vi "Fetch (NT Enum (Index).vi"(6 "default timestamp":timestamp, 7 "PV name":string, 8 "error in":errorcluster, 10 "default index":u16, 11 "Server in":refnum<class "Server.lvclass">) -> (0 "error out":errorcluster, 1 "PV found?":bool, 2 "index":u16, 3 "Server out":refnum<class "Server.lvclass">, 4 "timestamp":timestamp)   [LabVIEW 2020, in "PV Access.lvlib" / "PVA Server.lvlib" / "Server.lvclass"]
uses:
  Server.lvclass
  PV Data/PV Data/PV Data.lvclass
  Source/Source.lvclass
  Server.lvclass/Server.ctl
  PV Data/PV Data/Read Field (U16).vi
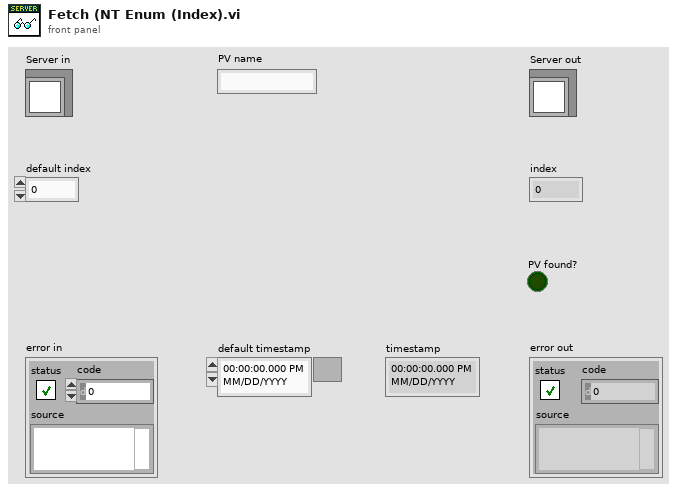
[diagram p1: front panel]
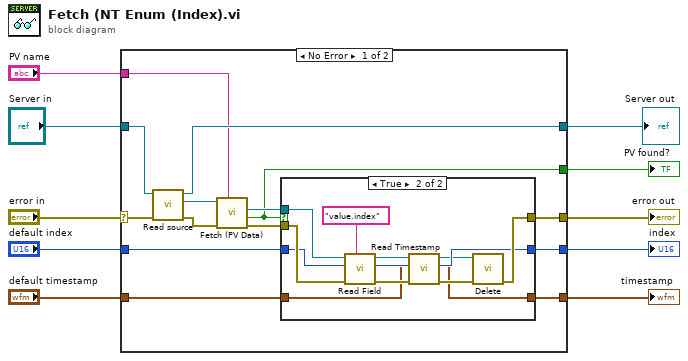
[diagram p0: block diagram]
diagram:
  n1 = case shown="No Error" "error in" {
    selector: "error in" -> [w12 w41]
    tunnel: [w17 w41] -> w10
    tunnel: "PV name" -> [w21 _]
    tunnel: "Server in" -> [w23 w43]
    tunnel: [w22 w43] -> w6
    tunnel: "default index" -> [w16 w42]
    tunnel: [w15 w42] -> w4
    tunnel: "default timestamp" -> [w14 w40]
    tunnel: [w13 w40] -> w2
    tunnel: [w11 _] -> w1
    frame No Error {
      n2 = call "Read source.vi"("error in (no error)"=w12, "Server in"=w23) -> ("error out"=w20:errorcluster, "Source"=w19:refnum<class "Source.lvclass">, "Server out"=w22:refnum<class "Server.lvclass">)  [unwired: 7 in]
      n3 = call "Fetch (PV Data).vi"("PV name"=w21, "error in"=w20, "Source in"=w19) -> ("error out"=w24:errorcluster, "PV found?"=w11:bool, "PV Data out"=w18:refnum<class "PV Data.lvclass">)  [unwired: 5 in, 1 out]
      n4 = case shown="True" w11 {
        tunnel: w24 -> [w26 w39]
        tunnel: w18 -> [_ w38]
        tunnel: [w26 w37] -> w17
        tunnel: w16 -> [w25 w36]
        tunnel: [w25 w32] -> w15
        tunnel: w14 -> [w27 w29]
        tunnel: [w27 w28] -> w13
        frame False {
        }
        frame True {
          n5 = call-poly "Read Field.vi"("field name"="value.index", "error in (no error)"=w39, "default"=w36, "PV Data in"=w38) -> ("error out"=w34:errorcluster, "value"=w32:u16, "PV Data out"=w33:refnum<class "PV Data.lvclass">)  [unwired: 5 in]
          n6 = call "Read Timestamp.vi"("error in"=w34, "timestamp in"=w29, "PV Data in"=w33) -> ("error out"=w30:errorcluster, "timestamp"=w28:timestamp, "PV Data out"=w31:refnum<class "PV Data.lvclass">)  [unwired: 5 in, 1 out]
          n7 = call "Delete.vi"("error in (no error)"=w30, "PV Data in"=w31) -> ("error out"=w37:errorcluster)  [unwired: 9 in]
        }
      }
    }
    frame Error {
    }
  }
  "Server out" <- w6
  "error out" <- w10
  "index" <- w4
  "timestamp" <- w2
  "PV found?" <- w1
